vi "BarbHeight (2).vi"(0 "Refnum in":T2, 1 "ROI Descriptor":T1 {"Contours"."Type" items=["No Selection", "Point", "Line", "Rectangle", "Oval", "Polygon", "Freehand Region", "Annulus", "Unused2", "Unused3", "Broken Line", "Freehand Line", "Rotated Rectangle"]}, 2 "Step Size":u32, 3 "Scan Direction":u16, 4 "Process":T3(ring), 5 "error in (no error)":errorcluster, 6 "Refnum in":T2, 7 "ROI Descriptor 2":T1 {"Contours"."Type" items=["No Selection", "Point", "Line", "Rectangle", "Oval", "Polygon", "Freehand Region", "Annulus", "Unused2", "Unused3", "Broken Line", "Freehand Line", "Rotated Rectangle"]}, 8 "Edge Options":T4 {"Edge Polarity" items=["All Edges", "Rising Edges", "Falling Edges"]; "Minimum Edge Strength" format="%.2f"; "Width" step=2; "Kernel Size" step=2}, 9 "Ta (Constant)":dbl, 10 "AvgMinMax":enum16{"Average", "Max", "Min"}(ring)) -> (14 "Numeric":dbl, 15 "Array":cluster{"X":sgl, "Y":sgl}[](array[cluster]), 16 "a":sgl, 17 "b":sgl, 18 "NumberOfIternations 2":i32, 19 "error out":errorcluster)   [LabVIEW 2015, in "Algorithm.lvclass"]
uses:
  Algorithm.lvclass
  <vilib>/vision/Image Controls.llb/IMAQ Image.ctl
  <vilib>/vision/Measure.llb/Edge Options.ctl
  <vilib>/vision/Measure.llb/Edge Polarity.ctl
  <vilib>/vision/NI_Vision_Development_Module.lvlib
panel:
  out "Numeric 3":i32
  out "Numeric 2":i32
  out "arccos(x)":sgl
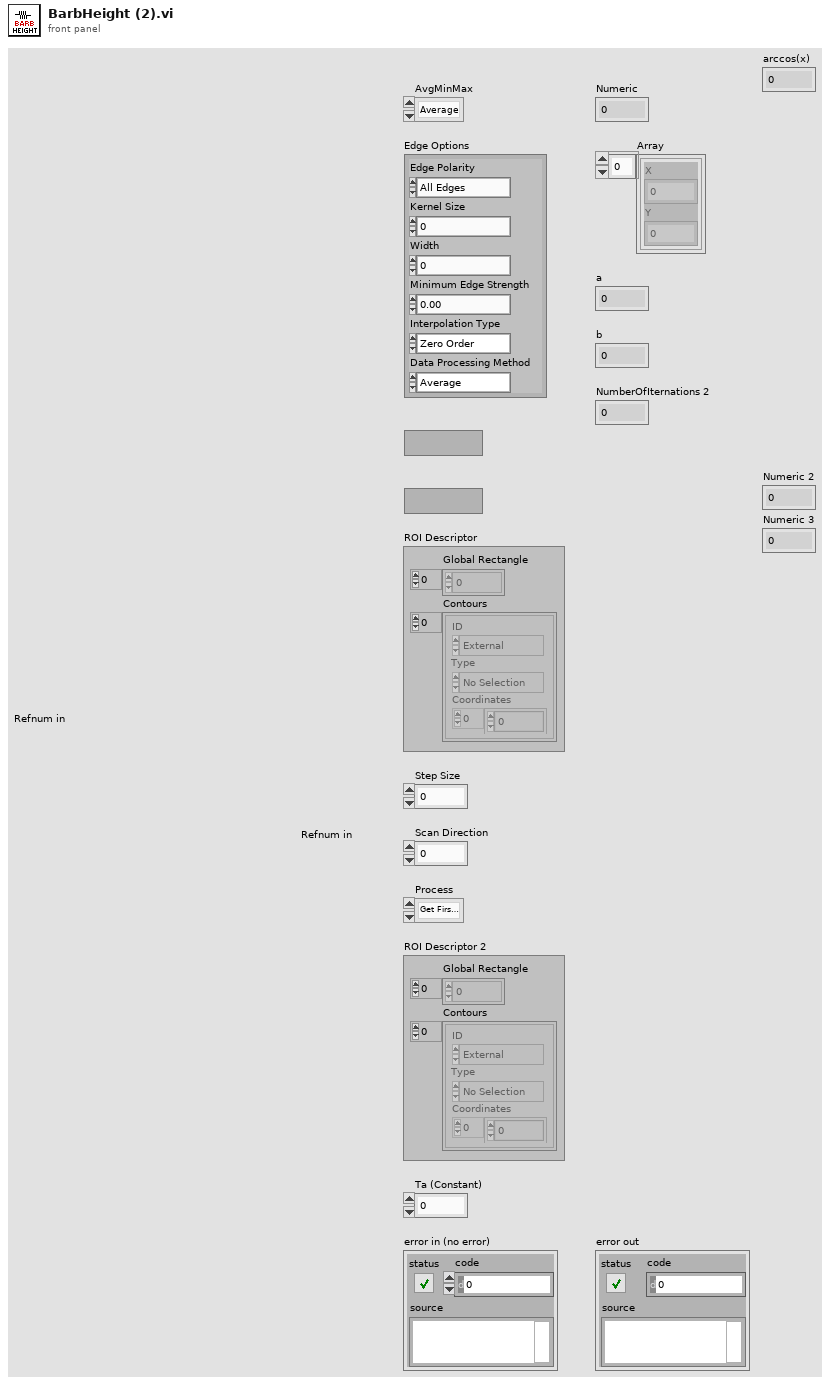
[diagram p1: front panel]
types:
  T1 = typedef "ROI Descriptor" = cluster{"Global Rectangle":i32[], "Contours":cluster{"ID":enum32{"External", "Internal"}, "Type":u32, "Coordinates":i32[]}[]}
  T2 = typedef "IMAQ Image.ctl" = refnum<image>
  T3 = enum16{"Get First Edge", "Get First + Last Edge", "Get All Edges", "Get Best Edge"}
  T4 = typedef "Edge Options.ctl" = cluster{"Edge Polarity":T5, "Kernel Size":u32, "Width":u32, "Minimum Edge Strength":sgl, "Interpolation Type":enum32{"Zero Order", "Bilinear", "Quadratic", "Cubic", "Bilinear Fixed"}, "Data Processing Method":enum32{"Average", "Median"}}
  T5 = typedef "Edge Polarity.ctl" = u32
  T6 = typedef "Edge New.ctl" = cluster{"Location (Pixel)":cluster{"X":sgl, "Y":sgl}, "Location (Real-World)":cluster{"X":sgl, "Y":sgl}, "Distance (Pixel)":dbl, "Distance (Real-World)":dbl, "Strength":dbl, "Noise":dbl, "Rising?":bool}
  T7 = typedef "Search Line.ctl" = cluster{"Start Point":cluster{"X":sgl, "Y":sgl}, "End Point":cluster{"X":sgl, "Y":sgl}, "Edge Info":T6[], "Edge Map":dbl[], "Calibration Valid":bool}
  T8 = cluster{"Center":cluster{"X":sgl, "Y":sgl}, "Major Axis":cluster{"Point 1":cluster{"X":sgl, "Y":sgl}, "Point 2":cluster{"X":sgl, "Y":sgl}}, "Minor Axis":cluster{"Point 1":cluster{"X":sgl, "Y":sgl}, "Point 2":cluster{"X":sgl, "Y":sgl}}}
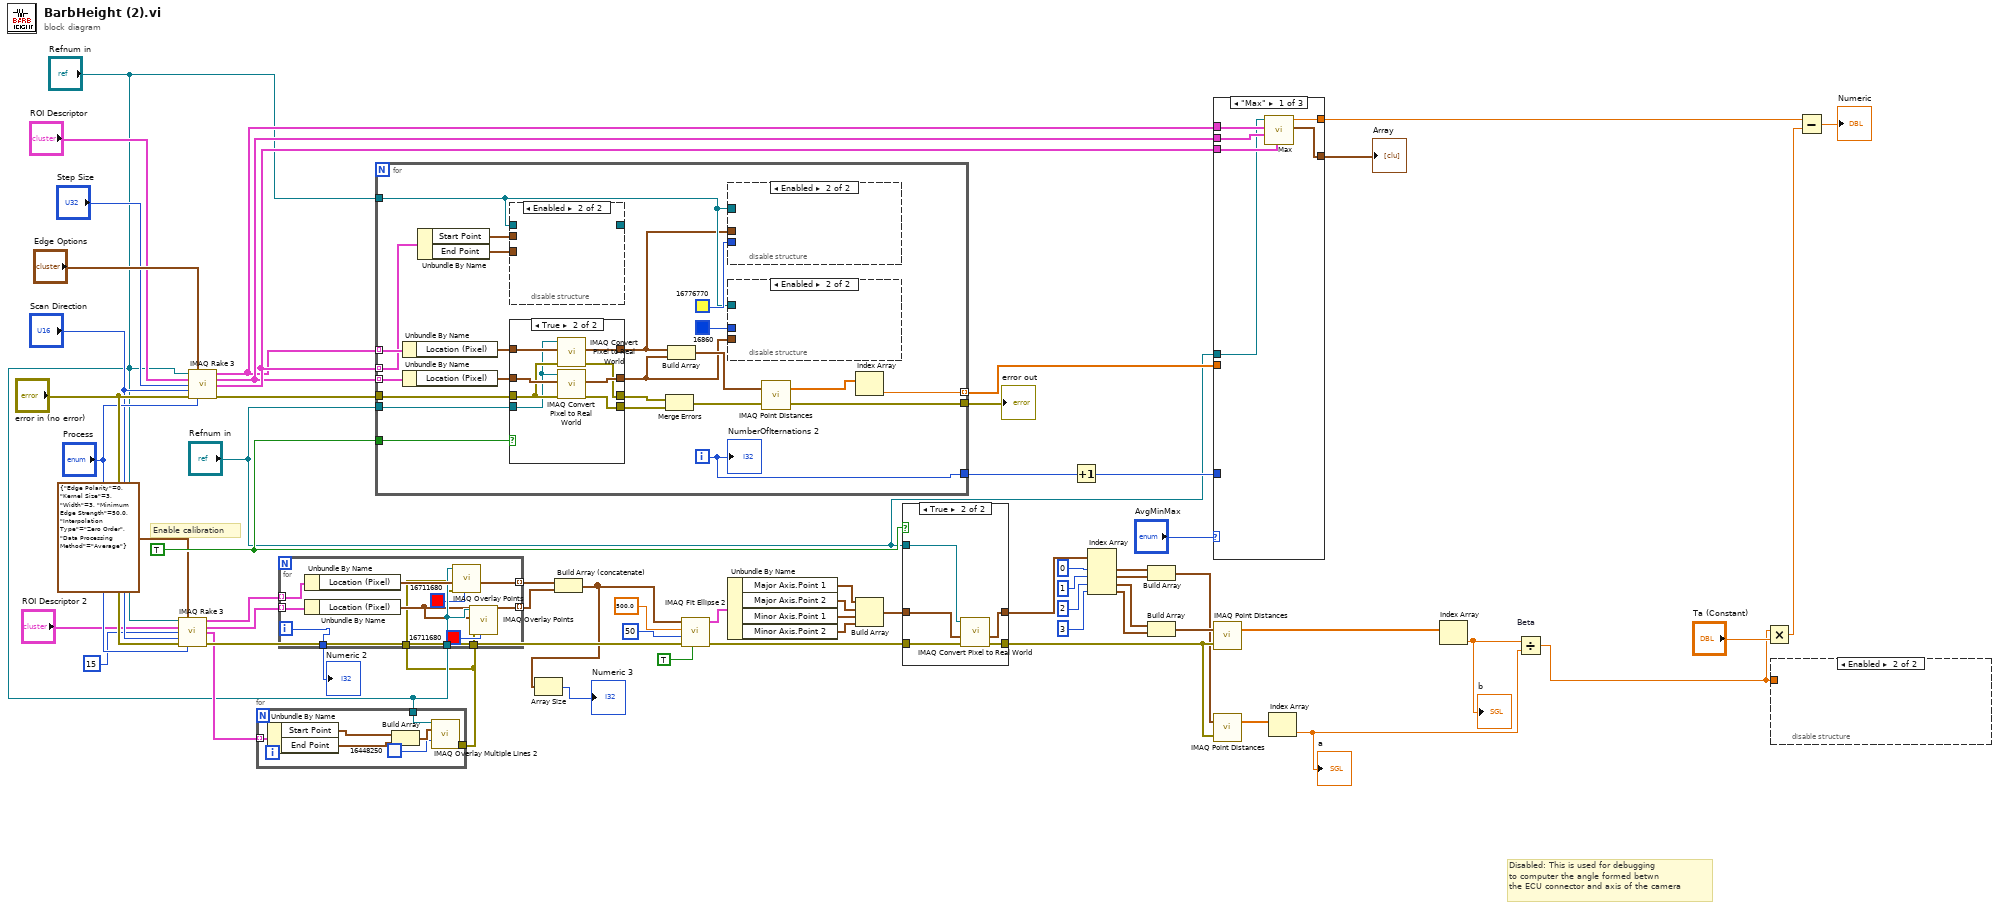
[diagram p0: block diagram]
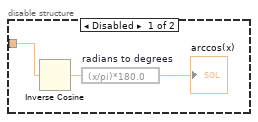
[diagram p2: hidden frame]
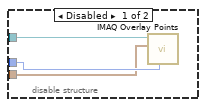
[diagram p7: hidden frame]
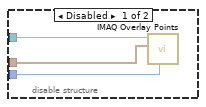
[diagram p8: hidden frame]
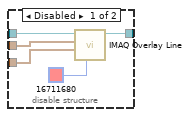
[diagram p9: hidden frame]
diagram:
  w14 = TRUE
  # "Disabled: This is used for debugging\nto computer the angle formed betwn\nthe ECU connector and axis of the camera"
  # "Enable calibration"
  n1 = call "IMAQ Rake 3"("Image"="Refnum in", "Edge Options"=T4 {"Edge Polarity"=0, "Kernel Size"=3, "Width"=3, "Minimum Edge Strength"=50.0, "Interpolation Type"=enum."Zero Order", "Data Processing Method"=enum."Average"}, "ROI Descriptor"="ROI Descriptor 2", "Step Size"=u32 15, "Scan Direction"="Scan Direction", "error in (no error)"="error in (no error)", "Process"="Process") -> ("First Edges"=w40:T6[], "Last Edges"=w41:T6[], "Search Lines"=w7:T7[], "error out"=w16:errorcluster)  [unwired: 5 in]
  n2 = call "IMAQ Rake 3"("Image"="Refnum in", "Edge Options"="Edge Options", "ROI Descriptor"="ROI Descriptor", "Step Size"="Step Size", "Scan Direction"="Scan Direction", "error in (no error)"="error in (no error)", "Process"="Process") -> ("First Edges"=w31:T6[], "Last Edges"=w32:T6[], "Search Lines"=w33:T7[], "error out"=w29:errorcluster)  [unwired: 5 in]
  n3 = for {
    tunnel: w7 -> [w70] mode=indexing
    tunnel: "Refnum in" -> [w66]
    tunnel: [w64] -> w5
    n4 = Unbundle By Name(w70) -> ("Start Point"=w69:cluster{"X":sgl, "Y":sgl}, "End Point"=w68:cluster{"X":sgl, "Y":sgl})
    n5 = Build Array(w69, w68) -> (w67:cluster{"X":sgl, "Y":sgl}[])
    n6 = call "IMAQ Overlay Multiple Lines 2"("Image"=w66, "Line End Points"=w67, "Color"=u32 16448250) -> ("error out"=w64:errorcluster)  [unwired: 11 in, 1 out]
  }
  n7 = for {
    tunnel: w40 -> [w80] mode=indexing
    tunnel: w41 -> [w79] mode=indexing
    tunnel: [w78] -> w42 mode=indexing
    tunnel: [w75] -> w43 mode=indexing
    tunnel: [w77] -> w8
    tunnel: "Refnum in" -> [w76]
    tunnel: w5 -> [w72]
    tunnel: w5 -> [w71]
    i -> [w77]
    n8 = Unbundle By Name(w80) -> ("Location (Pixel)"=w78:cluster{"X":sgl, "Y":sgl})
    n9 = Unbundle By Name(w79) -> ("Location (Pixel)"=w75:cluster{"X":sgl, "Y":sgl})
    n10 = call "IMAQ Overlay Points"("Color"=u32 16711680, "error in (no error)"=w71, "Image"=w76) -> ()  [unwired: 7 in, 2 out]
    n11 = call "IMAQ Overlay Points"("Color"=u32 16711680, "error in (no error)"=w72, "Point"=w75, "Image"=w76) -> ()  [unwired: 6 in, 2 out]
  }
  "Numeric 2" <- w8
  n12 = for {
    tunnel: "Refnum in" -> [w92]
    tunnel: w31 -> [w103] mode=indexing
    tunnel: w32 -> [w102] mode=indexing
    tunnel: w33 -> [w101] mode=indexing
    tunnel: [w95] -> w27 mode=indexing
    tunnel: [w96] -> w26
    tunnel: "Refnum in" -> [w87]
    tunnel: w29 -> [w86]
    tunnel: [w82] -> w30
    tunnel: w14 -> [w81]
    i -> [w96]
    n13 = Unbundle By Name(w103) -> ("Location (Pixel)"=w90:cluster{"X":sgl, "Y":sgl})
    n14 = Unbundle By Name(w102) -> ("Location (Pixel)"=w89:cluster{"X":sgl, "Y":sgl})
    n15 = Unbundle By Name(w101) -> ("Start Point"=w100:cluster{"X":sgl, "Y":sgl}, "End Point"=w99:cluster{"X":sgl, "Y":sgl})
    n16 = disable-structure shown="Enabled" {
      disable-tunnel: w100 -> [w125 _]
      disable-tunnel: w99 -> [w124 _]
      disable-tunnel: w92 -> [w123 _]
      disable-tunnel: [w122 _] -> _
      frame Disabled {
        n17 = call "IMAQ Overlay Line"("Color"=u32 16711680, "End Point"=w124, "Start Point"=w125, "Image"=w123) -> ("Image Out"=w122:T2)  [unwired: 6 in, 1 out]
      }
      frame Enabled {
      }
    }
    n18 = case shown="True" w81 {
      tunnel: [w106 w114] -> w91
      tunnel: w90 -> [w106 w113]
      tunnel: w89 -> [w105 w112]
      tunnel: [w105 w111] -> w88
      tunnel: w87 -> [_ w107]
      tunnel: w86 -> [w104 w110]
      tunnel: [w104 w109] -> w85
      tunnel: [w104 w108] -> w84
      frame False {
      }
      frame True {
        n19 = call "IMAQ Convert Pixel to Real World"("error in (no error)"=w110, "Pixel Coordinates"=w113, "Calibrated Image"=w107) -> ("error out"=w109:errorcluster, "Real World Coordinates"=w114:cluster{"X":sgl, "Y":sgl})  [unwired: 3 in, 4 out]
        n20 = call "IMAQ Convert Pixel to Real World"("error in (no error)"=w110, "Pixel Coordinates"=w112, "Calibrated Image"=w107) -> ("error out"=w108:errorcluster, "Real World Coordinates"=w111:cluster{"X":sgl, "Y":sgl})  [unwired: 3 in, 4 out]
      }
    }
    n21 = Merge Errors(w85, w84) -> (w83:errorcluster)
    n22 = Build Array(w91, w88) -> (w98:cluster{"X":sgl, "Y":sgl}[])
    n23 = disable-structure shown="Enabled" {
      disable-tunnel: u32 16776770 ("Color") -> [w120 _]
      disable-tunnel: w92 -> [w119 _]
      disable-tunnel: w91 -> [w118 _]
      frame Disabled {
        n24 = call "IMAQ Overlay Points"("Color"=w120, "Point"=w118, "Image"=w119) -> ()  [unwired: 7 in, 2 out]
      }
      frame Enabled {
      }
    }
    n25 = disable-structure shown="Enabled" {
      disable-tunnel: u32 16860 ("Color") -> [w117 _]
      disable-tunnel: w92 -> [w116 _]
      disable-tunnel: w88 -> [w115 _]
      frame Disabled {
        n26 = call "IMAQ Overlay Points"("Color"=w117, "Point"=w115, "Image"=w116) -> ()  [unwired: 7 in, 2 out]
      }
      frame Enabled {
      }
    }
    n27 = call "IMAQ Point Distances"("Points"=w98, "error in (no error)"=w83) -> ("Distances"=w97:sgl[], "error out"=w82:errorcluster)  [unwired: 3 in]
    n28 = Index Array(array=w97) -> (element=w95:sgl)  [unwired: 1 in]
    "NumberOfIternations 2" <- w96
  }
  "error out" <- w30
  n29 = Build Array (concatenate)(w42, w43) -> (w4:cluster{"X":sgl, "Y":sgl}[])
  n30 = Array Size(array=w4) -> (size(s)=→"Numeric 3":i32)
  n31 = call "IMAQ Fit Ellipse 2"("Reject Outliers (FALSE)"=TRUE, "error in (no error)"=w16, "Maximum Iterations"=50, "Minimum Score"=500.0, "Radial Points"=w4) -> ("error out"=w17:errorcluster, "Ellipse"=w22:T8)  [unwired: 1 in, 4 out]
  n32 = Unbundle By Name(w22) -> ("Major Axis.Point 1"=w21:cluster{"X":sgl, "Y":sgl}, "Major Axis.Point 2"=w20:cluster{"X":sgl, "Y":sgl}, "Minor Axis.Point 1"=w19:cluster{"X":sgl, "Y":sgl}, "Minor Axis.Point 2"=w18:cluster{"X":sgl, "Y":sgl})
  n33 = Build Array(w21, w20, w19, w18) -> (w47:cluster{"X":sgl, "Y":sgl}[])
  n34 = case shown="True" w14 {
    tunnel: [w126 w132] -> w56
    tunnel: [w127 w131] -> w48
    tunnel: w47 -> [w127 w130]
    tunnel: w17 -> [w126 w129]
    tunnel: "Refnum in" -> [_ w128]
    frame False {
    }
    frame True {
      n35 = call "IMAQ Convert Pixel to Real World"("error in (no error)"=w129, "Array of Pixel Coordinates"=w130, "Calibrated Image"=w128) -> ("error out"=w132:errorcluster, "Array of Real World Coordinates"=w131:cluster{"X":sgl, "Y":sgl}[])  [unwired: 3 in, 4 out]
    }
  }
  n36 = Increment(x=w26) -> (x+1=w25:i32)
  n37 = Index Array(array=w48, index #1=0 ("index"), index #2=1 ("index"), index #3=2 ("index"), index #4=3 ("index")) -> (element #1=w53:cluster{"X":sgl, "Y":sgl}, element #2=w54:cluster{"X":sgl, "Y":sgl}, element #3=w57:cluster{"X":sgl, "Y":sgl}, element #4=w58:cluster{"X":sgl, "Y":sgl})
  n38 = Build Array(w53, w54) -> (w55:cluster{"X":sgl, "Y":sgl}[])
  n39 = Build Array(w57, w58) -> (w59:cluster{"X":sgl, "Y":sgl}[])
  n40 = case shown="\"Max\"" "AvgMinMax" {
    tunnel: w25 -> [_ _ _]
    tunnel: [w134 _ _] -> w10
    tunnel: w27 -> [_ _ _]
    tunnel: w31 -> [w138 _ _]
    tunnel: w32 -> [w136 _ _]
    tunnel: w33 -> [w137 _ _]
    tunnel: [w135 _ _] -> w34
    tunnel: "Refnum in" -> [w133 _ _]
    frame "Max" {
      n41 = call "Max.vi"("Search Lines"=w137, "Last Edges"=w136, "First Edges"=w138, "Refnum in"=w133) -> ("Array"=w135:cluster{"X":sgl, "Y":sgl}[], "Numeric"=w134:sgl)  [unwired: 6 in]
    }
    frame "Min" {
    }
    frame "Average" {
    }
  }
  "Array" <- w34
  n42 = call "IMAQ Point Distances"("Points"=w59, "error in (no error)"=w56) -> ("Distances"=w61:sgl[])  [unwired: 3 in, 1 out]
  n43 = call "IMAQ Point Distances"("Points"=w55, "error in (no error)"=w56) -> ("Distances"=w60:sgl[])  [unwired: 3 in, 1 out]
  n44 = Index Array(array=w60) -> (element=w11:sgl)  [unwired: 1 in]
  "a" <- w11
  n45 = Index Array(array=w61) -> (element=w12:sgl)  [unwired: 1 in]
  "b" <- w12
  n46 = Divide "Beta"(x=w12, y=w11) -> (x/y=w9:sgl)
  n47 = Multiply(x=w9, y="Ta (Constant)") -> (x*y=w1:dbl)
  n48 = disable-structure shown="Enabled" {
    disable-tunnel: w9 -> [w141 _]
    frame Disabled {
      n49 = Inverse Cosine(1:w141) -> (0:w140:sgl)
      n50 = expression code="(x/pi)*180.0" "radians to degrees"(w140) -> (→"arccos(x)":sgl)
    }
    frame Enabled {
    }
  }
  n51 = Subtract(x=w10, y=w1) -> (x-y=→"Numeric":dbl)
